vi "PAN_extract_schedule.vi"(10 "command":string) -> (2 "schedule":T1[](array[typedef]))   [LabVIEW 2016]
uses:
  PAN_scheduler_element.ctl
panel:
  in  "action":T1
  out "millisecond timer value":u32
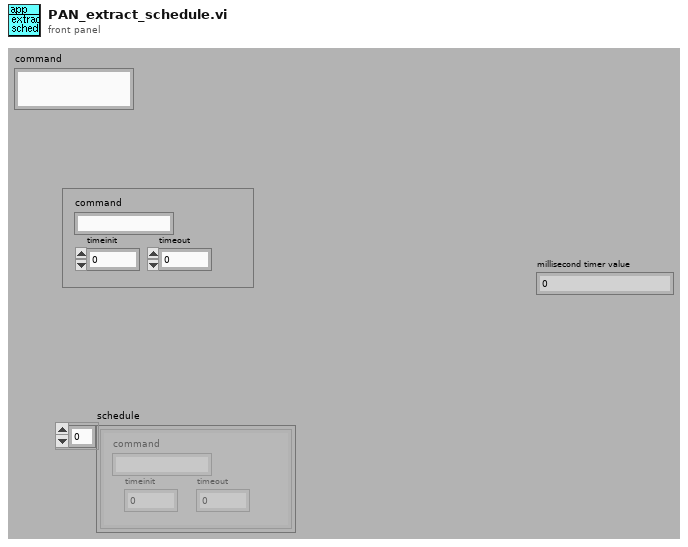
[diagram p1: front panel]
types:
  T1 = typedef "PAN_scheduler_element.ctl" = cluster{"command":string, "timeinit":i32, "timeout":i32}
  T2 = cluster{"second":i32, "minute":i32, "hour":i32, "day of month":i32, "month":i32, "year":i32, "day of week":i32, "day of year":i32, "is DST":i32}
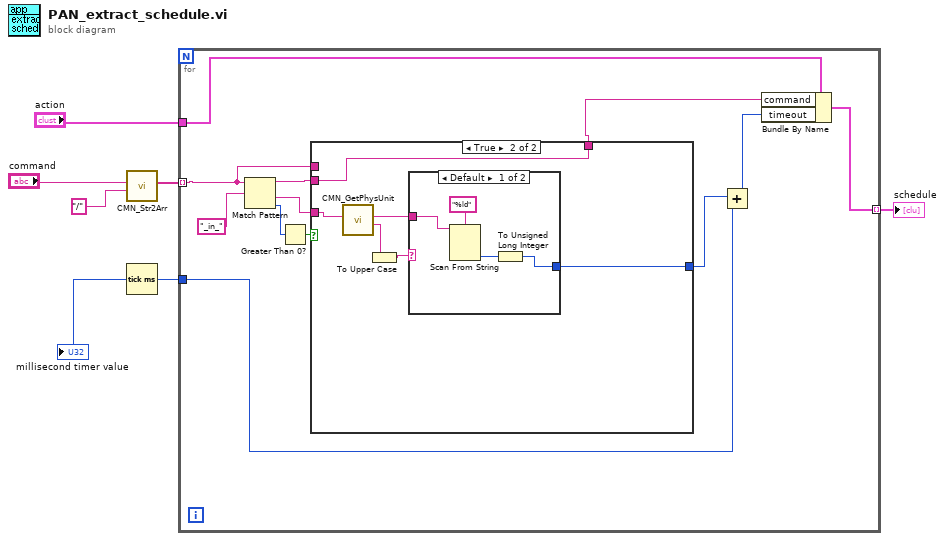
[diagram p0: block diagram]
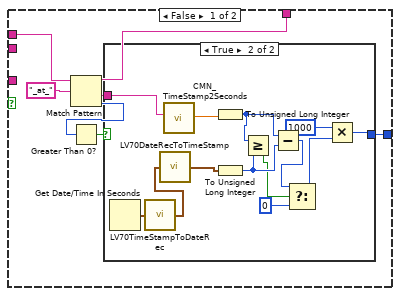
[diagram p2: hidden frame]
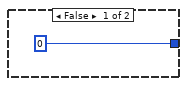
[diagram p3: hidden frame]
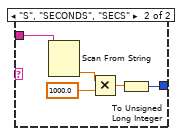
[diagram p4: hidden frame]
diagram:
  n1 = call "CMN_Str2Arr.vi"("separator"="/", "string in"="command") -> ("Array out"=w5:string[])  [unwired: 2 in, 7 out]
  n2 = Tick Count (ms)() -> (millisecond timer value=w4:u32)
  "millisecond timer value" <- w4
  n3 = for {
    tunnel: w5 -> [w12] mode=indexing
    tunnel: w4 -> [w14]
    tunnel: [w8] -> w3 mode=indexing
    tunnel: "action" -> [w10]
    n4 = Match Pattern(string=w12, regular expression="_in_") -> (before substring=w11:string, after substring=w15:string, offset past match=w16:i32)  [unwired: 2 out]
    n5 = Greater Than 0?(x=w16) -> (x > 0?=w17:bool)
    n6 = case shown="True" w17 {
      tunnel: w15 -> [_ w45]
      tunnel: [w25 w41] -> w13
      tunnel: w12 -> [w24 _]
      tunnel: w11 -> [_ w40]
      tunnel: [w20 w40] -> w7
      frame False {
        n7 = Match Pattern(string=w24, regular expression="_at_") -> (before substring=w20:string, after substring=w19:string, offset past match=w22:i32)  [unwired: 2 out]
        n8 = Greater Than 0?(x=w22) -> (x > 0?=w21:bool)
        n9 = case shown="True" w21 {
          tunnel: [u32 0 w28] -> w25
          tunnel: w19 -> [_ w39]
          frame False {
          }
          frame True {
            n10 = Get Date/Time In Seconds() -> (seconds since 1Jan1904=w27:timestamp)
            n11 = call <vilib>:"LV70TimeStampToDateRec.vi"("time stamp"=w27) -> ("date time rec"=w38:T2)
            n12 = call <vilib>:"LV70DateRecToTimeStamp.vi"("date time rec"=w38) -> ("Time Stamp"=w36:timestamp)
            n13 = call "CMN_TimeStamp2Seconds.vi"("TimeStamp string (yyyy-mm-ddThh:mm:ss)"=w39) -> ("seconds out"=w37:dbl)  [unwired: 1 in, 8 out]
            n14 = To Unsigned Long Integer(number=w37) -> (unsigned 32bit integer=w35:u32)
            n15 = To Unsigned Long Integer(number=w36) -> (unsigned 32bit integer=w34:u32)
            n16 = Greater Or Equal?(x=w35, y=w34) -> (x >= y?=w33:bool)
            n17 = Subtract(x=w35, y=w34) -> (x-y=w31:u32)
            n18 = Select(t=w31, s=w33, f=u32 0) -> (s? t:f=w30:u32)
            n19 = Multiply(x=u32 1000, y=w30) -> (x*y=w28:u32)
          }
        }
      }
      frame True {
        n20 = call "CMN_GetPhysUnit.vi"("command in"=w45) -> ("unit"=w43:string, "command out"=w44:string)  [unwired: 9 out]
        n21 = To Upper Case(1:w43) -> (0:w42:string)
        n22 = case shown="Default" w42 {
          tunnel: w44 -> [w49 w54]
          tunnel: [w46 w50] -> w41
          frame Default {
            n23 = Scan From String(format string="%ld", input string=w49) -> (output 1=w47:i32)  [unwired: 2 in, 4 out]
            n24 = To Unsigned Long Integer(number=w47) -> (unsigned 32bit integer=w46:u32)
          }
          frame "S", "SECONDS", "SECS" {
            n25 = Scan From String(input string=w54) -> (output 1=w53:dbl)  [unwired: 3 in, 4 out]
            n26 = Multiply(x=w53, y=1000.0) -> (x*y=w51:dbl)
            n27 = To Unsigned Long Integer(number=w51) -> (unsigned 32bit integer=w50:u32)
          }
        }
      }
    }
    n28 = Add(x=w13, y=w14) -> (x+y=w9:u32)
    n29 = Bundle By Name(cluster=w10, "command"=w7, "timeout"=w9) -> (w8:T1)
  }
  "schedule" <- w3
